vi "exec.vi"(8 "error in (no error)":errorcluster, 10 "context":refnum<class "Context.lvclass">, 11 "StartOpenLoopScan in":refnum<class "StartOpenLoopScan.lvclass">) -> (0 "error out":errorcluster, 2 "context 2":refnum<class "Context.lvclass">, 3 "StartOpenLoopScan out":refnum<class "StartOpenLoopScan.lvclass">)   [LabVIEW 2015, in "StartOpenLoopScan.lvclass"]
uses:
  StartOpenLoopScan.lvclass
  Context/Context.lvclass
  StartOpenLoopScan.lvclass/StartOpenLoopScan.ctl
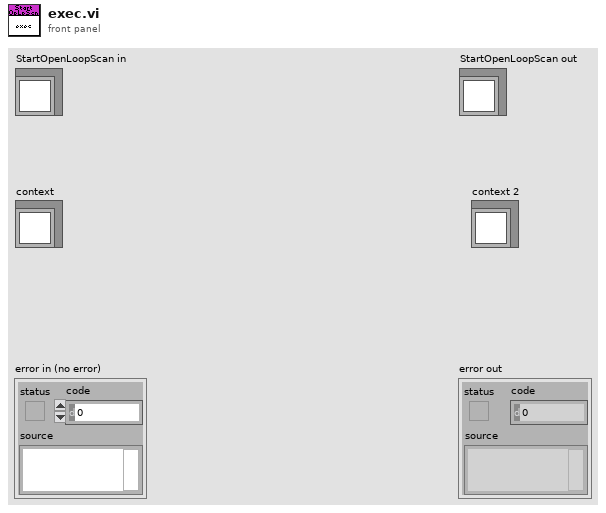
[diagram p1: front panel]
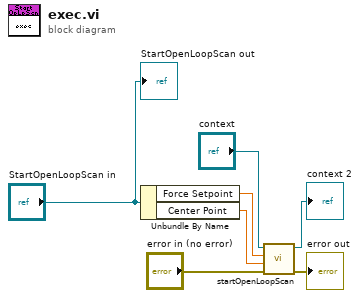
[diagram p0: block diagram]
diagram:
  n1 = Unbundle By Name("StartOpenLoopScan in") -> ("Force Setpoint"=w4:dbl[unit], "Center Point"=w3:dbl[unit])
  n2 = call "startOpenLoopScan.vi"("error in (no error)"="error in (no error)", "Center Point"=w3, "Force Setpoint"=w4, "Context in"="context") -> ("error out"=→"error out":errorcluster, "Context out"=→"context 2":refnum<class "Context.lvclass">)  [unwired: 6 in]
  "StartOpenLoopScan out" <- "StartOpenLoopScan in"
